vi "Get Step Result.vi"(8 "error in (no error)":errorcluster, 10 "Step ID":string, 11 "Execution in":refnum<class "Execution.lvclass">) -> (0 "error out":errorcluster, 1 "No Result?":bool, 2 "Result Status":string, 3 "Execution out":refnum<class "Execution.lvclass">)   [LabVIEW 2020, in "TSnax.lvlib" / "Execution.lvclass"]
uses:
  Execution.lvclass
  Execution.lvclass/Execution.ctl
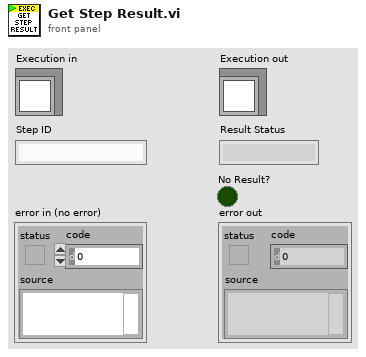
[diagram p1: front panel]
types:
  T1 = typedef "TSnax.lvlib/Execution.lvclass/Step Results.ctl" = cluster{"Map":map{string, string}}
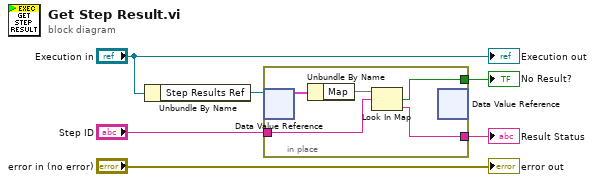
[diagram p0: block diagram]
diagram:
  n1 = Unbundle By Name("Execution in") -> ("Step Results Ref"=w5:refnum<data-value>)
  n2 = in-place {
    in-place-border: "Step ID" -> [w9]
    in-place-border: [w8] -> w2
    in-place-border: [w7] -> w1
    n3 = in-place-dvr #1(w5) -> (w11:T1)  [unwired: 1 out]
    n4 = Unbundle By Name(w11) -> ("Map"=w10:map{string, string})
    n5 = Look In Map(map=w10, key=w9) -> (key not found?=w7:bool, value=w8:string)  [unwired: 1 in]
    n6 = in-place-dvr #1() -> ()  [unwired: 1 in, 2 out]
  }
  "Result Status" <- w2
  "No Result?" <- w1
  "error out" <- "error in (no error)"
  "Execution out" <- "Execution in"
